vi "CpuLoadsOnly.vi"() -> ()   [LabVIEW 2019]
doc: "This VI runs in parallel to other tasks. It can contain as many user-defined periodic loops as you need. These can carry out PID or other sorts of timed response."
uses:
  <vilib>/NI_Real-Time Target Support.lvlib
panel:
  out "IndividualCpuLoads":dbl[](array[numeric]) format="%11.2f"
  out "Cpu Loads":dbl format="%11.2f"
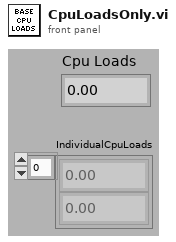
[diagram p1: front panel]
types:
  T1 = typedef "NI_Real-Time Target Support.lvlib/RT CPU Load.ctl" = cluster{"Total (%)":dbl, "Time Critical (%)":dbl, "Timed Structures (%)":dbl, "High (%)":dbl, "Above Normal (%)":dbl, "Normal (%)":dbl, "Background (%)":dbl, "Idle (%)":dbl, "ISR (%)":dbl}
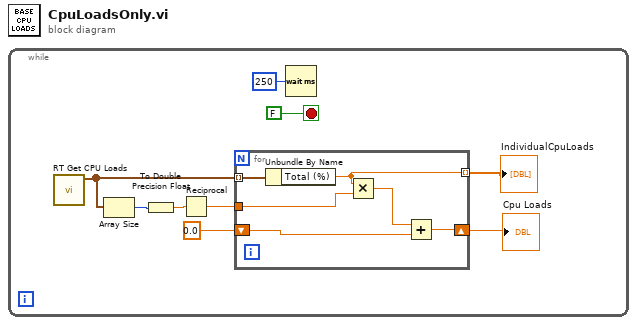
[diagram p0: block diagram]
diagram:
  n1 = while {
    stop <- FALSE stop-if-true
    n2 = call <vilib>:"RT Get CPU Loads.vi"() -> ("CPU loads"=w7:T1[])  [unwired: 10 in, 1 out]
    n3 = Array Size(array=w7) -> (size(s)=w6:i32)
    n4 = To Double Precision Float(number=w6) -> (double precision float=w5:dbl)
    n5 = Reciprocal(x=w5) -> (1/x=w4:dbl)
    n6 = for {
      tunnel: w7 -> [w15] mode=indexing
      tunnel: w4 -> [w14]
      shift-right: [w11] -> w1
      shift-left: 0.0 -> [w13]
      tunnel: [w10] -> w2 mode=indexing
      n7 = Unbundle By Name(w15) -> ("Total (%)"=w10:dbl)
      n8 = Multiply(x=w10, y=w14) -> (x*y=w12:dbl)
      n9 = Add(x=w12, y=w13) -> (x+y=w11:dbl)
    }
    "Cpu Loads" <- w1
    "IndividualCpuLoads" <- w2
    n10 = Wait (ms)(milliseconds to wait=u32 250) -> ()  [unwired: 1 out]
  }
